vi "getTemperature.vi"(6 "Channel":i32, 8 "error in (no error)":errorcluster, 11 "Instrument.Cryostat in":refnum<class "Instrument.Cryostat.lvclass">) -> (0 "error out":errorcluster, 1 "Status":string, 2 "Temperature (K)":dbl, 3 "Instrument.Cryostat out":refnum<class "Instrument.Cryostat.lvclass">, 4 "Finished?":bool)   [LabVIEW 2019, in "Instrument.Cryostat.lvclass"]
uses:
  Instrument.Cryostat.lvclass
  Instrument/Instrument.lvclass
  Typedefs/getTemperature--cluster.ctl
  7df5ea18-9fa6-471a-adc1-761ca2ff6fd2.vi
  C:/Users/patrick/Documents/GitHub/Instrument-Framework/lvsrc/Instrument/Instrument.lvclass
  C:/Program Files (x86)/National Instruments/LabVIEW 2019/vi.lib/JKI/JKI SMO/SMO/SMO.lvclass
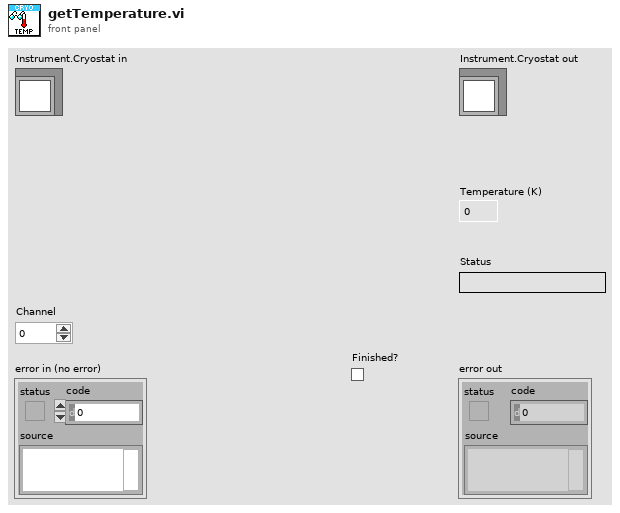
[diagram p1: front panel]
types:
  T1 = typedef "Instrument.Cryostat.lvclass/getTemperature--cluster.ctl" = cluster{"temperature":dbl, "status":string, "finished":bool}
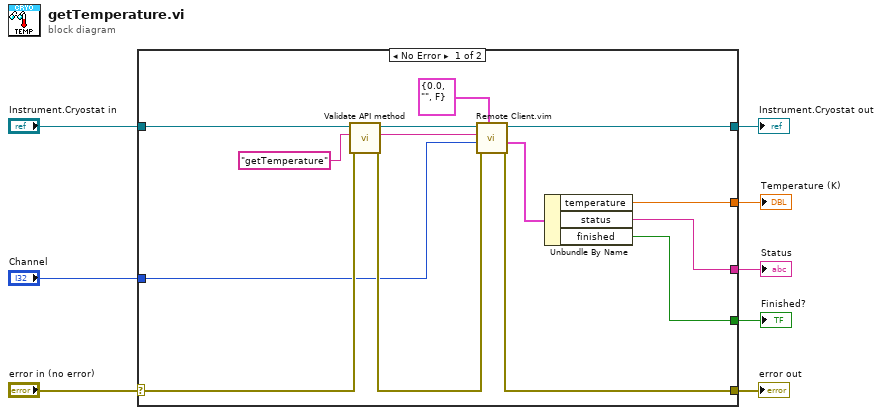
[diagram p0: block diagram]
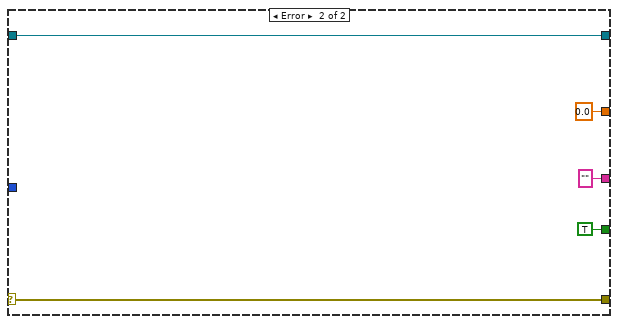
[diagram p2: hidden frame]
diagram:
  n1 = case shown="No Error" "error in (no error)" {
    selector: "error in (no error)" -> [w17 w27]
    tunnel: [w16 w27] -> w7
    tunnel: [w19 w26] -> w5
    tunnel: "Instrument.Cryostat in" -> [w20 w26]
    tunnel: [w13 0.0 ("Temperature (K)")] -> w4
    tunnel: [w12 "" ("Status")] -> w3
    tunnel: [w11 TRUE ("Finished?")] -> w2
    tunnel: "Channel" -> [w9 _]
    frame No Error {
      n2 = call "Validate API method.vi"("error in (no error)"=w17, "Command in"="getTemperature" ("error message (\"\")"), "Instrument in"=w20) -> ("error out"=w15:errorcluster, "command out"=w21:string, "Instrument out"=w18:refnum<class "Instrument.Cryostat.lvclass">)  [unwired: 6 in]
      n3 = call "Remote Client.vim"("Command out"=w21, "Data Out type"=T1 {"temperature"=0.0, "status"="", "finished"=FALSE} ("getTemperature"), "error in (no error)"=w15, "Data in"=w9, "Instrument in"=w18) -> ("error out"=w16:errorcluster, "Data out"=w10:T1, "Instrument out"=w19:refnum<class "Instrument.Cryostat.lvclass">)  [unwired: 4 in]
      n4 = Unbundle By Name(w10) -> ("temperature"=w13:dbl, "status"=w12:string, "finished"=w11:bool)
    }
    frame Error {
    }
  }
  "error out" <- w7
  "Instrument.Cryostat out" <- w5
  "Temperature (K)" <- w4
  "Status" <- w3
  "Finished?" <- w2
